vi "H5Gget_info_by_idx.vi"(3 "loc_id":i32, 4 "lapl_id":i32, 7 "group_name":string, 9 "error in (no error)":errorcluster) -> (0 "status":i32, 2 "group_info":T3 {"storage_type" items=["H5G_STORAGE_TYPE_UNKNOWN"=-1, "H5G_STORAGE_TYPE_SYMBOL_TABLE"=0, "H5G_STORAGE_TYPE_COMPACT"=1, "H5G_STORAGE_TYPE_DENSE"=2]}, 6 "error out":errorcluster)   [LabVIEW 2009]
uses:
  H5G_info_t.ctl
  H5G_storage_type_t.ctl
  H5_index_t.ctl
  H5_iter_order_t.ctl
  hdf5dll.dll
panel:
  in  "order":T1 items=["H5_ITER_UNKNOWN"=-1, "H5_ITER_INC"=0, "H5_ITER_DEC"=1, "H5_ITER_NATIVE"=2, "H5_ITER_N"=3]
  in  "index_type":T2 items=["H5_INDEX_UNKNOWN"=-1, "H5_INDEX_NAME"=0, "H5_INDEX_CRT_NAME"=1, "H5_INDEX_N"=2]
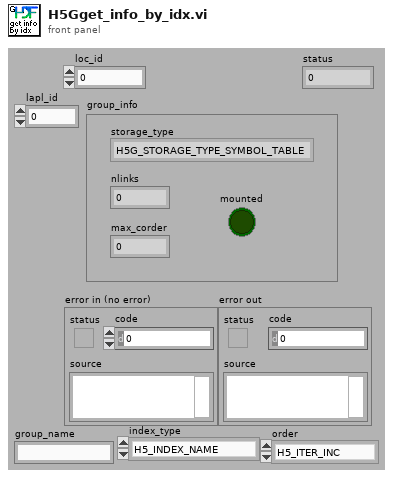
[diagram p1: front panel]
types:
  T1 = typedef "H5_iter_order_t.ctl" = i32
  T2 = typedef "H5_index_t.ctl" = i32
  T3 = typedef "H5G_info_t.ctl" = cluster{"storage_type":T4, "nlinks":i64, "max_corder":i64, "mounted":bool}
  T4 = typedef "H5G_storage_type_t.ctl" = i32
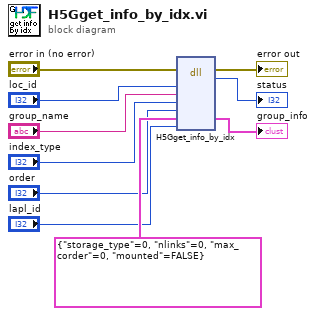
[diagram p0: block diagram]
diagram:
  n1 = dll-call lib="hdf5dll.dll" fn="H5Gget_info_by_idx"(error in="error in (no error)", "loc_id"="loc_id", "group_name"="group_name", "index_type"="index_type", "order"="order", "group_info"=T3 {"storage_type"=0, "nlinks"=0, "max_corder"=0, "mounted"=FALSE} ("H5G_info_t"), "lapl_id"="lapl_id") -> (error out=→"error out":errorcluster, "return type"=→"status":i32, "group_info"=→"group_info":T3)  [unwired: 7 in, 1 out]
